vi "Drivetrain.vi"   [LabVIEW 2012]
uses:
  <vilib>/Rock Robotics/WPI/Solenoid/WPI_SolenoidValue.ctl
  Robot Global Data.vi
  <vilib>/Rock Robotics/WPI/Solenoid/WPI_SolenoidSetEnum.vi
  <vilib>/Rock Robotics/WPI/RobotDrive/WPI_RobotDriveGetSetRefNum.vi
types:
  T1 = typedef "WPI_SolenoidValue.ctl" = enum16{"Off", "On", "Forward", "Reverse"}
  T2 = typedef "WPI_SolenoidDevRef.ctl" = cluster{"DevStatus":errorcluster, "Solenoid Module":T3, "Forward Solenoid Channel":T4, "Reverse Solenoid Channel":T4}
  T3 = typedef "FPGA_TypedefSolenoidModule.ctl" = enum16{"Solenoid Module 1", "Solenoid Module 2"}
  T4 = typedef "WPI_SolenoidChannel.ctl" = enum8{"Solenoid 1", "Solenoid 2", "Solenoid 3", "Solenoid 4", "Solenoid 5", "Solenoid 6", "Solenoid 7", "Solenoid 8", "Invalid"}
  T5 = typedef "WPI_RobotDriveDevRef.ctl" = cluster{"DevStatus":errorcluster, "Motors[]":T6[], "Square Inputs":bool, "Max Output":dbl, "Isochronous":bool}
  T6 = typedef "WPI_MotorControlDeviceRef.ctl" = cluster{"DeviceStatus":errorcluster, "Type":enum16{"PWM", "CAN"}, "PWM":cluster{"Digital Module":T7, "PWM Channel":T8, "DeadBand":T9}, "CAN":cluster{"Device Number":u8, "Control Mode":T10, "Semaphore":T11, "Max Vout":dbl}, "Invert":bool, "TransformRef":T12, "InvTransformRef":T12}
  T7 = typedef "FPGA_TypedefDigitalModule.ctl" = enum16{"Digital Module 1", "Digital Module 2"}
  T8 = typedef "FPGA_DIOPWMChannel.ctl" = enum8{"PWM 1", "PWM 2", "PWM 3", "PWM 4", "PWM 5", "PWM 6", "PWM 7", "PWM 8", "PWM 9", "PWM 10", "Invalid"}
  T9 = typedef "WPI_PWMDeadband.ctl" = cluster{"Name":string, "maxPositivePwm":i32, "minPositivePwm":i32, "centerPwm":i32, "maxNegativePwm":i32, "minNegativePwm":i32, "angularRange":u16}
  T10 = typedef "WPI_CANJaguar_ControlMode.ctl" = enum8{"Percent VBus", "Current", "Speed", "Position", "Voltage"}
  T11 = typedef "Semaphore RefNum" = refnum<k1>
  T12 = typedef "WPI_PWMTransform_ConPane.ctl" = refnum<vi>
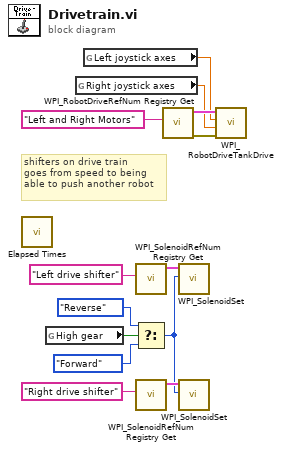
[diagram p0: block diagram]
diagram:
  # "shifters on drive train\ngoes from speed to being\nable to push another robot"
  n1 = call "Elapsed Times.vi"() -> ()  [unwired: 3 in, 1 out]
  n2 = global read "Robot Global Data.vi" "High gear"() -> (w8:bool)
  n3 = global read "Robot Global Data.vi" "Right joystick axes"() -> (w9:dbl)
  n4 = global read "Robot Global Data.vi" "Left joystick axes"() -> (w11:dbl)
  n5 = call <vilib>:"WPI_SolenoidRefNum Registry Get.vi"("refnum name"="Left drive shifter") -> ("SolenoidDevRef"=w1:T2)  [unwired: 9 in, 1 out]
  n6 = Select(t=WPI_SolenoidValue."Reverse" ("Value"), s=w8, f=WPI_SolenoidValue."Forward") -> (s? t:f=w3:T1)
  n7 = call <vilib>:"WPI_SolenoidRefNum Registry Get.vi"("refnum name"="Right drive shifter") -> ("SolenoidDevRef"=w6:T2)  [unwired: 9 in, 1 out]
  n8 = call <vilib>:"WPI_RobotDriveRefNum Registry Get.vi"("refnum name"="Left and Right Motors") -> ("error out"=w10:errorcluster, "RobotDriveDevRef"=w13:T5)  [unwired: 1 in, 8 out]
  n9 = call-poly <vilib>:"WPI_SolenoidSet.vi"("Value"=w3, "SolenoidDevRef"=w1) -> ()  [unwired: 8 in, 2 out]
  n10 = call-poly <vilib>:"WPI_SolenoidSet.vi"("Value"=w3, "SolenoidDevRef"=w6) -> ()  [unwired: 8 in, 2 out]
  n11 = call <vilib>:"WPI_RobotDriveTankDrive.vi"("error in (no error)"=w10, "Right axis value"=w9, "Left axis value"=w11, "RobotDriveDevRef"=w13) -> ()  [unwired: 5 in, 3 out]
